vi "Release Control Cluster.vi"(11 "output cluster":T1={"I-O.lvclass"=refnum, "Gantry"=refnum, "Dispenser"="COM1"}) -> ()   [LabVIEW 2020, in "Controller.lvclass"]
uses:
  Controller.lvclass
  I-O/I-O.lvclass
  Controllers.ctl
  C:/Program Files (x86)/Aerotech/A3200/LabVIEW/2010/Bin/Aerotech.A3200.dll
  Program Files (x86)/Aerotech/A3200/LabVIEW/2010/Bin/Aerotech.A3200.dll
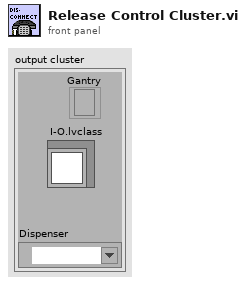
[diagram p1: front panel]
types:
  T1 = typedef "Controller.lvclass/Controllers.ctl" = cluster{"I-O.lvclass":refnum<class "I-O.lvclass">, "Gantry":refnum<k24>, "Dispenser":refnum<visa-resource-name>}
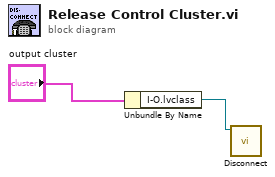
[diagram p0: block diagram]
diagram:
  n1 = Unbundle By Name("output cluster") -> ("I-O.lvclass"=w1:refnum<class "I-O.lvclass">)
  n2 = call-dynamic "Disconnect.vi"("I-O in"=w1) -> ()  [unwired: 9 in, 1 out]
